vi "KE6220 -- Get Arm Layer Trig Layer Params.vi"(0 "Resource In":refnum<visa-resource-name>, 1 "Check For SCPI Errors? (T)":bool=TRUE, 11 "error in (no error)":errorcluster) -> (4 "Resource Out (dupl)":refnum<visa-resource-name>, 8 "6220 Arm Trig Params":T1={"Arm Layer Input Trig Bypassed?"=FALSE, "Arm Layer Input Trig Source"=enum."Immediate", "Arm Layer Input Trig Link Line"=enum."1", "Arm Layer Input Trig Timer Interval (s)"=0.001, "Arm Layer Output Trig Mode"=enum."No Trig Out", "Arm Layer Output Trig Link Line"=enum."1", "Trig Layer Input Trig Source"=enum."Immediate", "Trig Layer Input Trig Link Line"=enum."1", "Trig Layer Output Trig Mode"=enum."No Trig Out", "Trig Layer Output Trig Link Line"=enum."1"} {"Arm Layer Input Trig Timer Interval (s)" min=0.001 max=99999.999 step=0.001 format="%.3f"}, 15 "error out":errorcluster)   [LabVIEW 2010, in "Keithley 622x.lvlib"]
doc: "Returns the parameters for the 'Arm' and 'Trigger' layers of the trigger model. Note that this VI can be used with both the 6220 and 6221, but it is really intended for use with the 6220, since there is a corresponding VI for the 6221."
uses:
  Keithley 622x.lvlib
  Low Level/Typedefs/KE622x -- Trig Source.ctl
  Low Level/Typedefs/KE622x -- Trig Link Line.ctl
  Low Level/Typedefs/KE622x -- Trig Output Mode.ctl
  Low Level/Typedefs/KE622x -- Arm Source.ctl
  Low Level/Typedefs/KE622x -- Arm Output Mode.ctl
  Low Level/Typedefs/KE622x -- Arm Timer Interval.ctl
  Typedefs/KE6220 -- Arm Trig Params.ctl
panel:
  # "Arm Layer"
  # "Trig Layer"
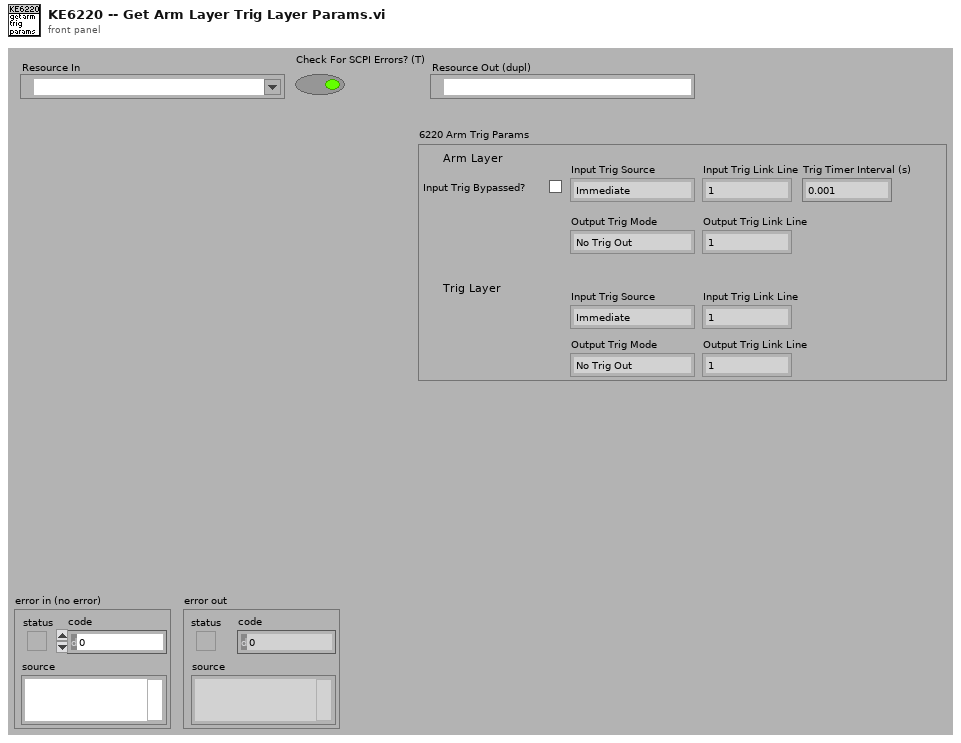
[diagram p1: front panel]
types:
  T1 = typedef "Keithley 622x.lvlib/KE6220 -- Arm Trig Params.ctl" = cluster{"Arm Layer Input Trig Bypassed?":bool, "Arm Layer Input Trig Source":T2, "Arm Layer Input Trig Link Line":T3, "Arm Layer Input Trig Timer Interval (s)":T4, "Arm Layer Output Trig Mode":T5, "Arm Layer Output Trig Link Line":T3, "Trig Layer Input Trig Source":T6, "Trig Layer Input Trig Link Line":T3, "Trig Layer Output Trig Mode":T7, "Trig Layer Output Trig Link Line":T3}
  T2 = typedef "Keithley 622x.lvlib/KE622x -- Arm Source.ctl" = enum16{"Immediate", "Bus (*TRG)", "Timer", "Manual", "Trigger Link", "SOT Falling Edge", "SOT Rising Edge", "SOT Either Edge"}
  T3 = typedef "Keithley 622x.lvlib/KE622x -- Trig Link Line.ctl" = enum16{"1", "2", "3", "4", "5", "6"}
  T4 = typedef "Keithley 622x.lvlib/KE622x -- Arm Timer Interval.ctl" = dbl
  T5 = typedef "Keithley 622x.lvlib/KE622x -- Arm Output Mode.ctl" = enum16{"No Trig Out", "Trig Out On Enter Arm", "Trig Out On Exit Arm"}
  T6 = typedef "Keithley 622x.lvlib/KE622x -- Trig Source.ctl" = enum16{"Immediate", "Trigger Link"}
  T7 = typedef "Keithley 622x.lvlib/KE622x -- Trig Output Mode.ctl" = enum16{"No Trig Out", "Source Turn On", "After Source Delay"}
  T8 = typedef "Keithley 622x.lvlib/KE622x -- Arm Layer Params.ctl" = cluster{"Bypass Arm Layer\nInput Trigger?":bool, "Input Trig Source":T2, "Input Trig Link Line":T3, "Arm Timer Interval (s)":T4, "Output Trig Mode":T5, "Output Trig Link Line":T3}
  T9 = typedef "Keithley 622x.lvlib/KE622x -- Trig Layer Params.ctl" = cluster{"Input Trig Source":T6, "Input Trig Link Line":T3, "Output Trig Mode":T7, "Output Trig Link Line":T3}
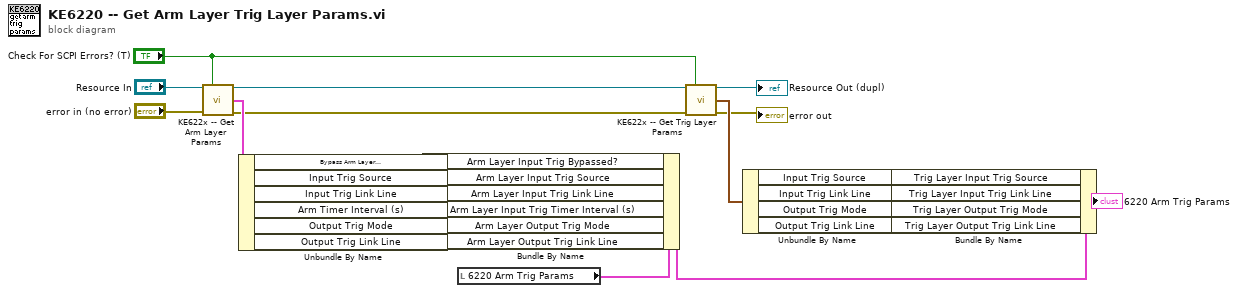
[diagram p0: block diagram]
diagram:
  n1 = call "KE622x -- Get Arm Layer Params.vi"("Resource In"="Resource In", "Check For SCPI Errors? (T)"="Check For SCPI Errors? (T)", "error in (no error)"="error in (no error)") -> ("Resource Out (dupl)"=w12:refnum<visa-resource-name>, "Arm Params"=w19:T8, "error out"=w11:errorcluster)  [unwired: 10 in]
  n2 = Unbundle By Name(w19) -> ("Bypass Arm Layer\nInput Trigger?"=w18:bool, "Input Trig Source"=w17:T2, "Input Trig Link Line"=w16:T3, "Arm Timer Interval (s)"=w15:T4, "Output Trig Mode"=w14:T5, "Output Trig Link Line"=w13:T3)
  n3 = local read "6220 Arm Trig Params"() -> (w20:T1)
  n4 = Bundle By Name(cluster=w20, "Arm Layer Input Trig Bypassed?"=w18, "Arm Layer Input Trig Source"=w17, "Arm Layer Input Trig Link Line"=w16, "Arm Layer Input Trig Timer Interval (s)"=w15, "Arm Layer Output Trig Mode"=w14, "Arm Layer Output Trig Link Line"=w13) -> (w10:T1)
  n5 = call "KE622x -- Get Trig Layer Params.vi"("Resource In"=w12, "Check For SCPI Errors? (T)"="Check For SCPI Errors? (T)", "error in (no error)"=w11) -> ("Resource Out (dupl)"=→"Resource Out (dupl)":refnum<visa-resource-name>, "Trig Layer Params"=w9:T9, "error out"=→"error out":errorcluster)  [unwired: 10 in]
  n6 = Unbundle By Name(w9) -> ("Input Trig Source"=w8:T6, "Input Trig Link Line"=w7:T3, "Output Trig Mode"=w6:T7, "Output Trig Link Line"=w5:T3)
  n7 = Bundle By Name(cluster=w10, "Trig Layer Input Trig Source"=w8, "Trig Layer Input Trig Link Line"=w7, "Trig Layer Output Trig Mode"=w6, "Trig Layer Output Trig Link Line"=w5) -> (→"6220 Arm Trig Params":T1)
